vi "retrieveStandardOutput.vi"(8 "error in (no error)":errorcluster, 9 "control name (stdout)":string="stdout", 11 "VI in":refnum<vi>) -> (0 "error out":errorcluster, 2 "stdout":string, 3 "VI out":refnum<vi>)   [LabVIEW 2013, in "openCronJob.lvlib" / "Job.StaticVIRef.lvclass"]
uses:
  Job.StaticVIRef.lvclass
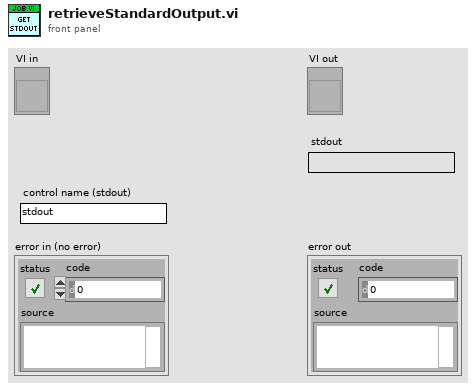
[diagram p1: front panel]
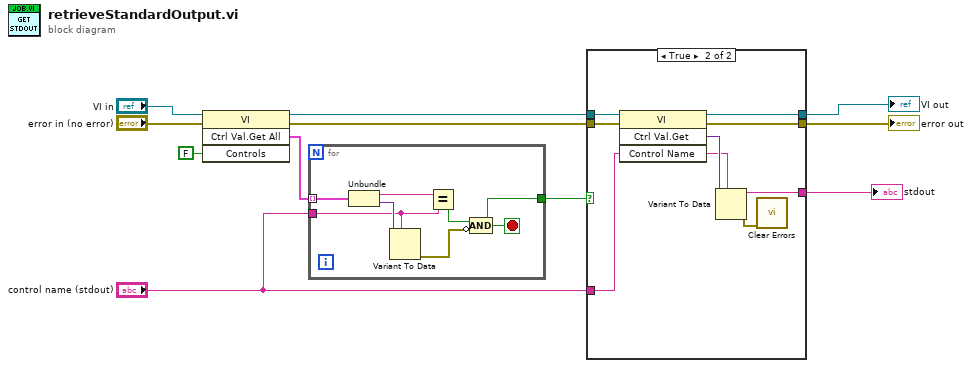
[diagram p0: block diagram]
diagram:
  n1 = invoke class="VI" method="Ctrl Val.Get All"(reference="VI in", error in="error in (no error)", "Controls"=FALSE) -> (reference out=w7:refnum<vi>, error out=w5:errorcluster, "Get All Control Values Variant"=w3:cluster{"Name":string, "Variant Data":variant}[])  [unwired: 1 in, 1 out]
  n2 = for {
    tunnel: w3 -> [w18] mode=indexing
    tunnel: "control name (stdout)" -> [w15]
    tunnel: [w12] -> w1
    stop <- w12 stop-if-true
    n3 = Unbundle(w18) -> ("Name"=w16:string, "Variant Data"=w17:variant)
    n4 = Variant To Data(type=w15, Variant=w17) -> (error out=w13:errorcluster)  [unwired: 1 in, 1 out]
    n5 = Equal?(x=w16, y=w15) -> (x = y?=w14:bool)
    n6 = Compound Arithmetic op=AND(w14, invert w13) -> (w12:bool)
  }
  n7 = case shown="True" w1 {
    tunnel: [w19 w28] -> w11
    tunnel: [w20 w27] -> w10
    tunnel: w7 -> [w20 w26]
    tunnel: w5 -> [w19 w25]
    tunnel: [_ w22] -> w4
    tunnel: "control name (stdout)" -> [_ w23]
    frame False {
    }
    frame True {
      n8 = invoke class="VI" method="Ctrl Val.Get"(reference=w26, error in=w25, "Control Name"=w23) -> (reference out=w27:refnum<vi>, error out=w28:errorcluster, "Get Control Value Variant"=w24:variant)  [unwired: 1 in, 1 out]
      n9 = Variant To Data(type=w23, Variant=w24) -> (data=w22:string, error out=w21:errorcluster)  [unwired: 1 in]
      n10 = call <vilib>:"Clear Errors.vi"("error in (no error)"=w21) -> ()  [unwired: 6 in, 1 out]
    }
  }
  "error out" <- w11
  "VI out" <- w10
  "stdout" <- w4
